vi "Read Reason.vi"(8 "error in (no error)":errorcluster, 11 "Rejected Future in":refnum<class "Rejected Promise.lvclass">) -> (0 "error out":errorcluster, 2 "Reason":errorcluster, 3 "Rejected Future out":refnum<class "Rejected Promise.lvclass">)   [LabVIEW 2017, in "Promise.lvlib" / "Rejected Promise.lvclass"]
uses:
  Rejected Promise.lvclass
  Rejected Promise.lvclass/Rejected Promise.ctl
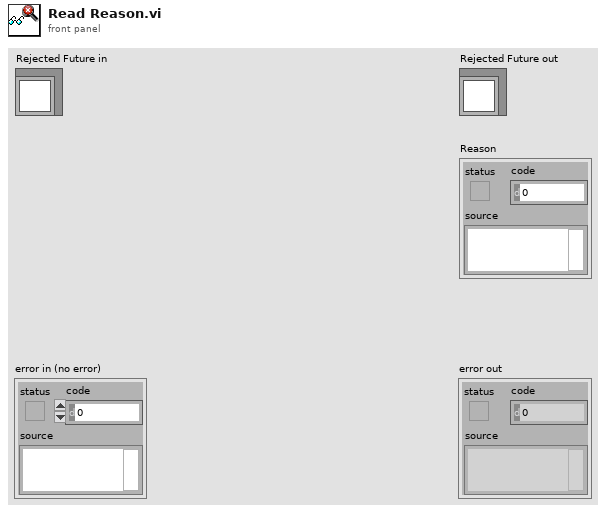
[diagram p1: front panel]
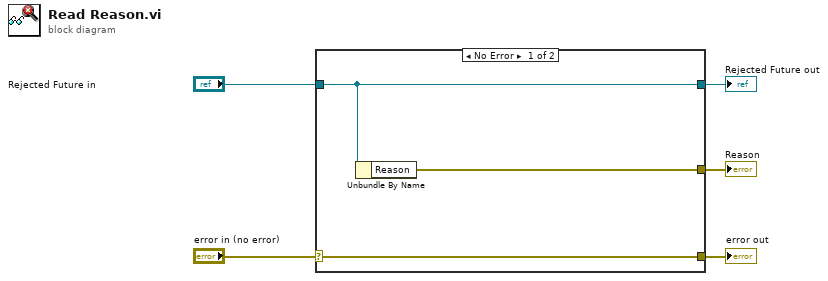
[diagram p0: block diagram]
diagram:
  n1 = case shown="No Error" "error in (no error)" {
    selector: "error in (no error)" -> [w8 w9]
    tunnel: [w8 w9] -> w4
    tunnel: [w7 w10] -> w2
    tunnel: "Rejected Future in" -> [w7 w10]
    tunnel: [w6 _] -> w1
    frame No Error {
      n2 = Unbundle By Name(w7) -> ("Reason"=w6:errorcluster)
    }
    frame Error {
    }
  }
  "error out" <- w4
  "Rejected Future out" <- w2
  "Reason" <- w1
